vi "Sub_online_LEMP_Update.vi"(0 "Prior Eigenvalues":dbl[](array[numeric]), 5 "Prior Eigenvectors Squared":T1, 7 "1/deltaStiff":dbl, 9 "Mode count":i32, 11 "Effected dof":i32) -> (4 "Updated Eigenvalues":dbl[](array[numeric]))   [LabVIEW 2019]
uses:
  <vilib>/Analysis/Matrix/Datatypes/RealMatrix.ctl
  secular_solver/bin/Debug1/secular_solver.dll
  <vilib>/Analysis/Matrix/NI_Matrix.lvlib
panel:
  # "Inputs"
  # "Output"
  # "This Vi the minimal possible operations to prep data for the secular equation solver, then sails to \"C\" to use the secular equation solver dll and returns the updated Eigenvalues. While offline, the prior Eigenvalues, the squares of each value in the prior Eigenvectors the equivalent stiffness change for the rolle are each attained. The modes used and the Effected DOF are constants provided at runtime. The index and  truncation operations are miniscules time uses however \"technically\" if memory and speed are absolutely critical then truncation of the eigenvalues and eigenvectors could be performed at initialization losing the modecount \"dynamic\" variation at runtime functionality. The memory time and memory saved is O(n+n*(n-m)) where n is the number of nodes and m is the number of modes.\n\n              - Alexander Vereen AFRL Summer scholars 2022"
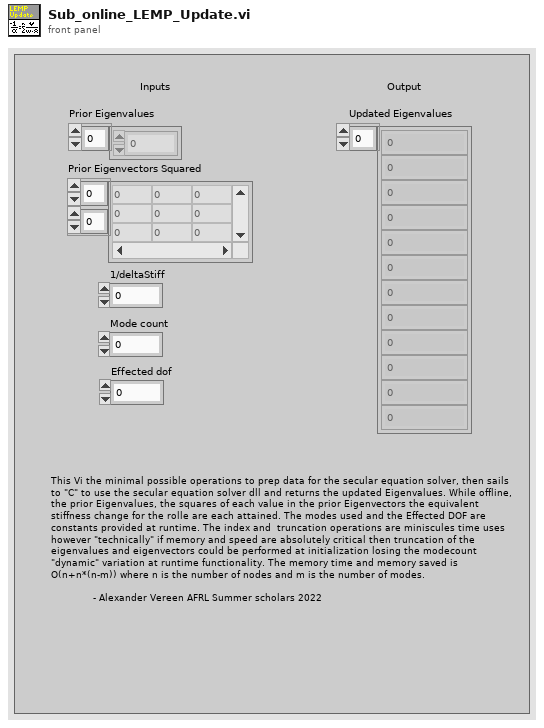
[diagram p1: front panel]
types:
  T1 = typedef "NI_Matrix.lvlib/RealMatrix.ctl" = dbl[][]
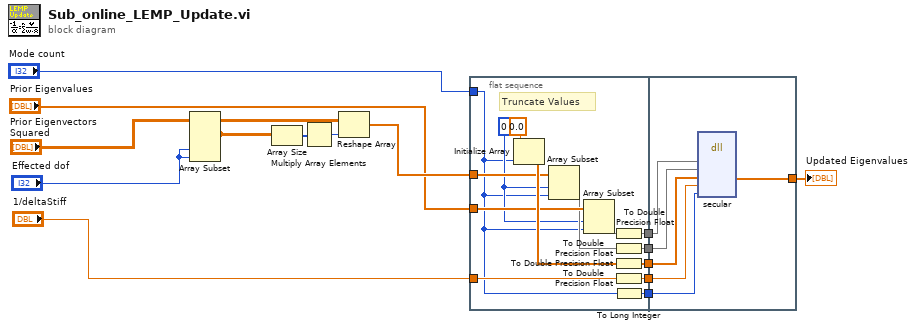
[diagram p0: block diagram]
diagram:
  n1 = Array Subset(array="Prior Eigenvectors Squared", index (col)="Effected dof", length (col)="Effected dof") -> (w7:T1)  [unwired: 2 in]
  n2 = Array Size(array=w7) -> (size(s)=w10:i32[])
  n3 = Multiply Array Elements(1:w10) -> (0:w9:i32)
  n4 = Reshape Array(w7, w9) -> (w8:dbl[])
  n5 = flat-sequence {
    tunnel: w8 -> [w26]
    tunnel: "Prior Eigenvalues" -> [w25]
    tunnel: "1/deltaStiff" -> [w29]
    tunnel: "Mode count" -> [w20]
    tunnel: [w21] -> w15
    tunnel: [w19] -> w14
    tunnel: [w17] -> w12
    tunnel: [w18] -> w11
    tunnel: [w16] -> w13
    tunnel: w15 -> [w35]
    tunnel: w14 -> [w34]
    tunnel: w13 -> [w33]
    tunnel: w12 -> [w32]
    tunnel: w11 -> [w31]
    tunnel: [w30] -> w6
    frame #0 {
      w23 = 0
      # "Truncate Values"
      n6 = Initialize Array(0.0, w20) -> (w27:dbl[])
      n7 = Array Subset(array=w26, index=w23, length=w20) -> (w24:dbl[])
      n8 = Array Subset(array=w25, index=w23, length=w20) -> (w22:dbl[])
      n9 = To Double Precision Float(number=w22) -> (double precision float=w21:dbl[])
      n10 = To Double Precision Float(number=w24) -> (double precision float=w19:dbl[])
      n11 = To Double Precision Float(number=w27) -> (double precision float=w18:dbl[])
      n12 = To Double Precision Float(number=w29) -> (double precision float=w17:dbl)
      n13 = To Long Integer(number=w20) -> (32bit integer=w16:i32)
    }
    frame #1 {
      n14 = dll-call lib="C:/Users/PXIe-8880/Documents/AFRL_summer_2022/LabVIEW_FEA_simulation_2022/Main_code/secular_solver/bin/Debug1/secular_solver.dll" fn="secular"("d"=w35, "v"=w34, "sol"=w31, "p"=w32, "mode"=w33) -> ("sol"=w30:dbl[])  [unwired: 8 in, 2 out]
    }
  }
  "Updated Eigenvalues" <- w6
